vi "Stop Actor.vi"(8 "error in (no error)":errorcluster, 11 "StopEnabledActor in":refnum<class "StopEnabledActor.lvclass">) -> (0 "error out":errorcluster, 3 "StopEnabledActor out":refnum<class "StopEnabledActor.lvclass">)   [LabVIEW 2017, in "StopEnabledActor.lvclass"]
uses:
  StopEnabledActor.lvclass
  StopEnabledActor.lvclass/StopEnabledActor.ctl
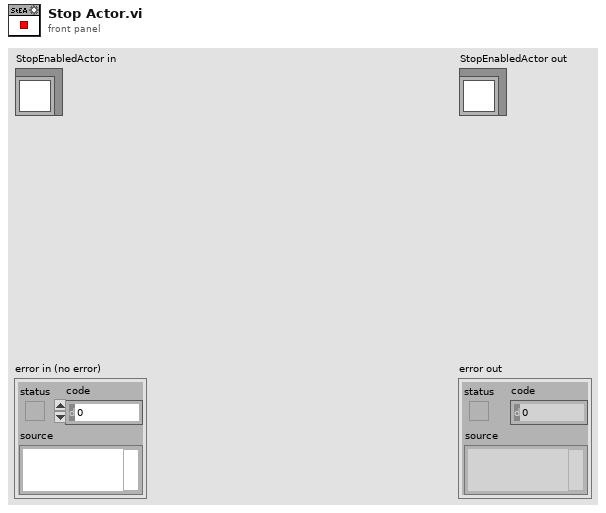
[diagram p1: front panel]
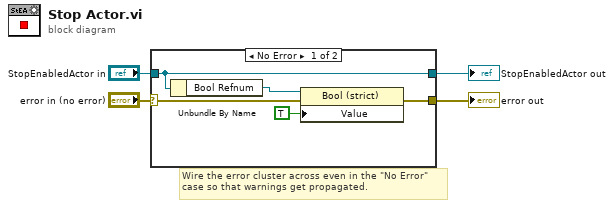
[diagram p0: block diagram]
diagram:
  # "Wire the error cluster across even in the \"No Error\"\ncase so that warnings get propagated."
  n1 = case shown="No Error" "error in (no error)" {
    selector: "error in (no error)" -> [w9 w11]
    tunnel: [w7 w11] -> w3
    tunnel: [w8 w10] -> w1
    tunnel: "StopEnabledActor in" -> [w8 w10]
    frame No Error {
      n2 = Unbundle By Name(w8) -> ("Bool Refnum"=w6:refnum<vi>)
      n3 = property class="Bool (strict)"(reference=w6, error in=w9, "Value"=TRUE) -> (error out=w7:errorcluster)  [unwired: 1 out]
    }
    frame Error {
    }
  }
  "error out" <- w3
  "StopEnabledActor out" <- w1
